vi "Initialize.vi"(8 "error in (no error)":errorcluster, 11 "userinfo file":path) -> (0 "error out":errorcluster, 3 "[User] Userinfo Binary out":refnum<class "[User] Userinfo Binary.lvclass">)   [LabVIEW 2020, in "[User] Userinfo Binary.lvclass"]
uses:
  [User] Userinfo Binary.lvclass
  [User] Userinfo Binary.lvclass/[User] Userinfo Binary.ctl
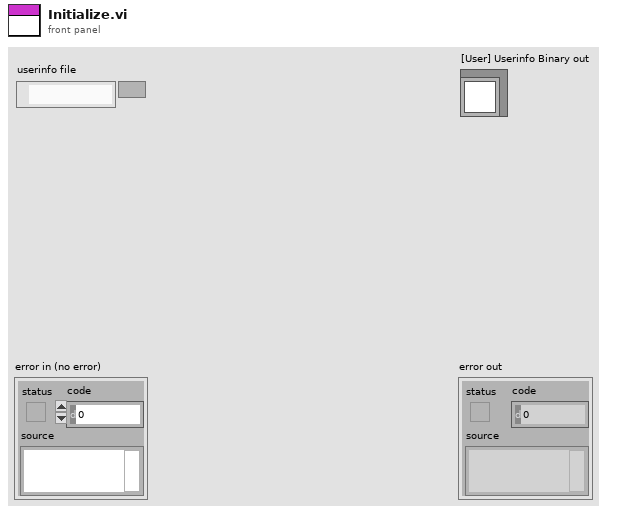
[diagram p1: front panel]
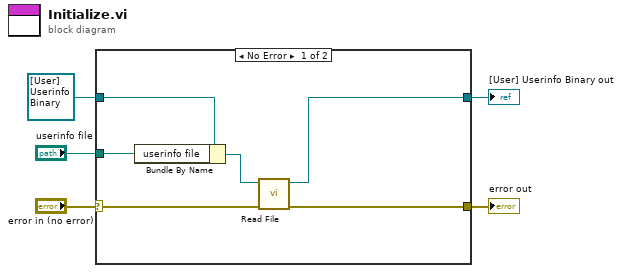
[diagram p0: block diagram]
diagram:
  n1 = case shown="No Error" "error in (no error)" {
    selector: "error in (no error)" -> [w9 w13]
    tunnel: [w7 w13] -> w1
    tunnel: refnum<class "[User] Userinfo Binary.lvclass"> refnum ("[User] Userinfo Binary in") -> [w11 w12]
    tunnel: [w6 w12] -> w2
    tunnel: "userinfo file" -> [w10 _]
    frame No Error {
      n2 = Bundle By Name(cluster=w11, "userinfo file"=w10) -> (w8:refnum<class "[User] Userinfo Binary.lvclass">)
      n3 = call "Read File.vi"("error in (no error)"=w9, "[User] Userinfo Binary in"=w8) -> ("error out"=w7:errorcluster, "[User] Userinfo Binary out"=w6:refnum<class "[User] Userinfo Binary.lvclass">)  [unwired: 8 in]
    }
    frame Error {
    }
  }
  "error out" <- w1
  "[User] Userinfo Binary out" <- w2
